vi "getValue.vi"(8 "error in (no error)":errorcluster, 11 "tBSONObjectID in":refnum<class "tBSONObjectID.lvclass">) -> (0 "error out":errorcluster, 2 "Value":string, 3 "tBSONObjectID out":refnum<class "tBSONObjectID.lvclass">)   [LabVIEW 2013, in "BSON.lvlib" / "tBSONObjectID.lvclass"]
uses:
  tBSONObjectID.lvclass
  tBSONObjectID.lvclass/tBSONObjectID.ctl
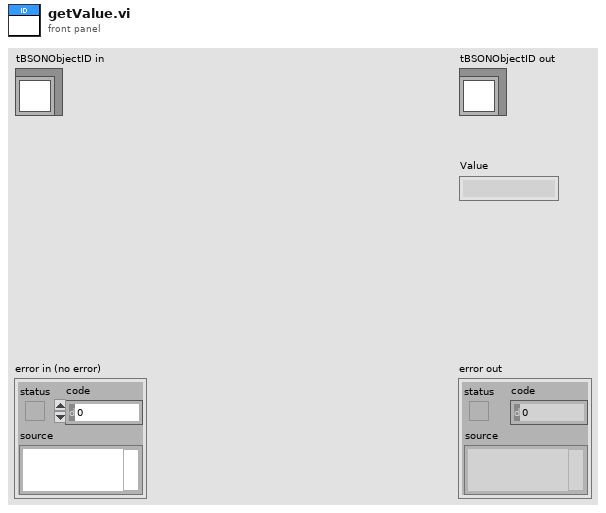
[diagram p1: front panel]
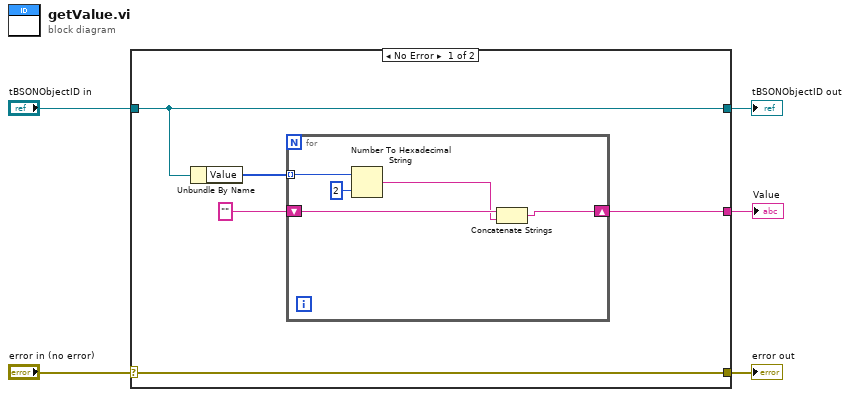
[diagram p0: block diagram]
diagram:
  n1 = case shown="No Error" "error in (no error)" {
    selector: "error in (no error)" -> [w7 w17]
    tunnel: [w7 w17] -> w4
    tunnel: [w10 w16] -> w2
    tunnel: "tBSONObjectID in" -> [w10 w16]
    tunnel: [w6 _] -> w1
    frame No Error {
      n2 = Unbundle By Name(w10) -> ("Value"=w8:u8[])
      n3 = for {
        shift-right: [w12] -> w6
        shift-left: "" -> [w14]
        tunnel: w8 -> [w15] mode=indexing
        n4 = Number To Hexadecimal String(1:i16 2 ("width (-)"), 2:w15) -> (0:w13:string)
        n5 = Concatenate Strings(w14, w13) -> (w12:string)
      }
    }
    frame Error {
    }
  }
  "error out" <- w4
  "tBSONObjectID out" <- w2
  "Value" <- w1
